vi "getCurrent.vi"(8 "error in (no error)":errorcluster, 10 "Channel Nr (1)":string="1", 11 "VISA resource name":refnum<visa-resource-name>) -> (0 "error out":errorcluster, 2 "Current im Amps":dbl=1.0 format="%#_13g", 3 "VISA resource name out":refnum<visa-resource-name>)   [LabVIEW 2023, in "Tti-Pl303Qmd.lvlib"]
doc: "Get Current of Channel"
uses:
  Tti-Pl303Qmd.lvlib
  <vilib>/Utility/error.llb/Error Cluster From Error Code.vi
  <vilib>/ErrorRing/Error Ring.xnode
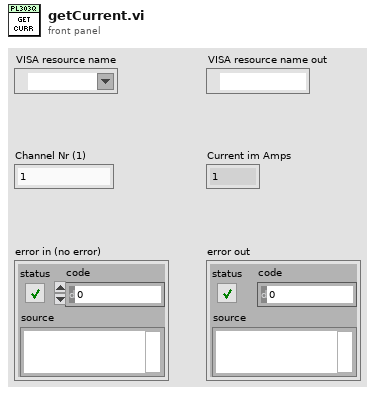
[diagram p1: front panel]
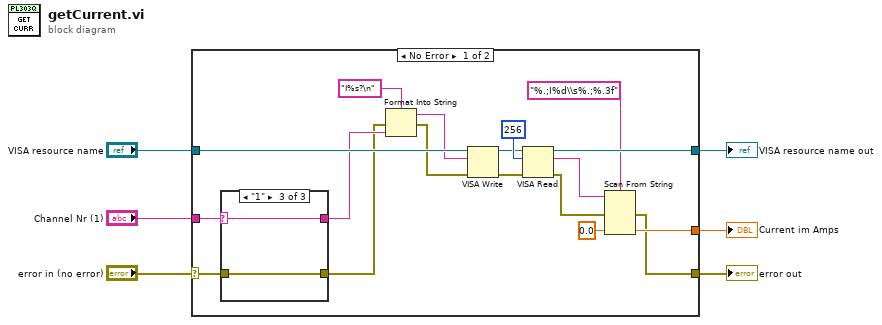
[diagram p0: block diagram]
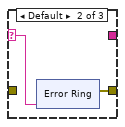
[diagram p3: hidden frame]
diagram:
  n1 = case shown="No Error" "error in (no error)" {
    selector: "error in (no error)" -> [w22 w39]
    tunnel: "VISA resource name" -> [w24 w38]
    tunnel: [w8 w39] -> w2
    tunnel: "Channel Nr (1)" -> [w23 _]
    tunnel: [w14 w38] -> w3
    tunnel: [w10 _] -> w1
    frame No Error {
      n2 = case shown="\"1\"" w23 {
        selector: w23 -> [w26 w27 w36]
        tunnel: w22 -> [w25 _ w37]
        tunnel: [w25 w28 w37] -> w19
        tunnel: [w26 _ w36] -> w20
        frame "2" {
        }
        frame Default {
          n3 = xnode "Error Ring"("parameter 0"=w27) -> ("error out"=w28:errorcluster)
        }
        frame "1" {
        }
      }
      n4 = Format Into String(format string="I%s?\n" ("write buffer"), error in=w19, w20) -> (resulting string=w17:string, error out=w18:errorcluster)  [unwired: 1 in]
      n5 = VISA Write(VISA resource name=w24, write buffer=w17, error in (no error)=w18) -> (VISA resource name out=w13:refnum<visa-resource-name>, error out=w16:errorcluster)  [unwired: 1 out]
      n6 = VISA Read(VISA resource name=w13, byte count=u32 256, error in (no error)=w16) -> (VISA resource name out=w14:refnum<visa-resource-name>, read buffer=w12:string, error out=w9:errorcluster)  [unwired: 1 out]
      n7 = Scan From String(format string="%.;I%d\\s%.;%.3f", input string=w12, error in=w9, default 2=0.0 ("default value 2")) -> (error out=w8:errorcluster, output 2=w10:dbl)  [unwired: 3 in, 2 out]
    }
    frame Error {
    }
  }
  "error out" <- w2
  "Current im Amps" <- w1
  "VISA resource name out" <- w3
